vi "Format Log Entry.vi"(3 "Log Entry":T1) -> (1 "Entry String":string)   [LabVIEW 2020, in "GPackTools.lvlib" / "GPackCLI.lvclass"]
uses:
  GPackCLI.lvclass
  CLILogger/Log Entry.ctl
  CLILogger/CLILogger.lvclass
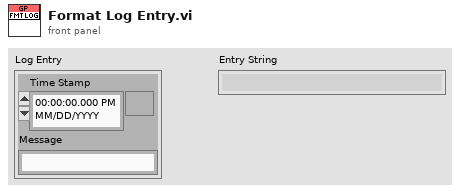
[diagram p1: front panel]
types:
  T1 = typedef "GPackTools.lvlib/CLILogger.lvclass/Log Entry.ctl" = cluster{"Time Stamp":timestamp, "Message":string}
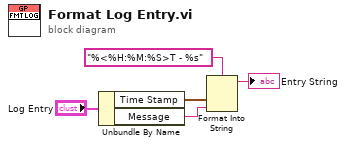
[diagram p0: block diagram]
diagram:
  n1 = Unbundle By Name("Log Entry") -> ("Time Stamp"=w3:timestamp, "Message"=w2:string)
  n2 = Format Into String(format string="%<%H:%M:%S>T - %s", w3, w2) -> (resulting string=→"Entry String":string)  [unwired: 2 in, 1 out]
